vi "Parse CSV String.vi"(7 "delimiter (,)":string=",", 10 "error in":errorcluster, 11 "CSV string":string) -> (2 "error out":errorcluster, 3 "2-D array":string[][](array[string]))   [LabVIEW 2020, in "infolib.lvlib"]
doc: "<b>http://en.wikipedia.org/wiki/Comma-separated_values</b>\n\nConvert a CSV (Character Separated Values) spreadsheet string to a 2D array of strings.\nThe input CSV spreadsheet string is assumed to be ANSI encoded and formatted in accordance with RFC-4180 (see <b>http://tools.ietf.org/html/rfc4180</b>). \nAll escaped double quotes will be un-escaped in the output array.\n\nRev. 0.4.0 2017-03-01 updated for infostr - removed replacing of EOLS by LF and opening/closing quotes by straight quotes\n\nRev 0.3.0 02/20/2014 Ryan Porter\n- Added feature to replace all EOLs (0x0A, 0x0D) with LF (0x0A) so as to avoid adding a blank row when encountering CR+LF at the end of a line.\n- Added feature to allow any single character delimiter (not just the comma).\n- Removed the read text file and path terminals. \n- Changed Icon and connector pane layout.\n- Added error case structure around diagram.\n- Changed file name to Parse CSV String\n\nRev 0.2.0 06/08/2011 P. Brooks\n Added feature to replace opening and closing double quotes (0x93 & 0x94) with simple quote (0x22).\n\nRev 0.1.0 05/31/2011 P. Brooks\n Added option to handle strings. If CSV string is NULL (default) then the file in CSV File Path will be parsed instead of CSV string.\n\nRev 0.0.0 05/09/2011 P. Brooks\n Originated."
uses:
  infolib.lvlib
  <vilib>/Utility/error.llb/whitespace.ctl
panel:
  # "Parse CSV String.vi\n\nConvert a CSV (Character Separated Values) spreadsheet string to a 2D array of strings.\nThe input CSV spreadsheet string is assumed to be ANSI encoded and formatted in accordance with RFC-4180 (see http://tools.ietf.org/html/rfc4180). \nAll EOLs (CR, LF or CRLF) will be converted to LF and all escaped double quotes will be un-escaped in the output array."
  # "Wikipedia Example Text \n(using opening and closing quotes)"
  # "Year,Make,Model,Description,Price\n1997,Ford,E350, “ac, abs, moon”,3000.00\n1999,Chevy,“Venture ““Extended Edition”””,“”,4900.00\n1999,Chevy,“ Venture ““ Extended Edition, Very Large”””,“”,5000.00\n1996,Jeep,Grand Cherokee,“MUST SELL!\nair, moon roof, loaded”,4799.00"
  # "http://en.wikipedia.org/wiki/Comma-separated_values"
  # "Robust CSV v1.1.0\n\nCopyright © 2014, Ryan Porter\nAll rights reserved.\n\nAuthor:\t Ryan Porter\nLAVA Name: Porter\nContact Info:\tContact via PM on lavag.org\n\nLabVIEW Versions:\nLV 2013 (Windows)\nLV 2012 (Windows)\nLV 8.6 (Windows)\n\nDependencies:\nLAVA Palette\n\nDescription:\nThis package contains VIs for reading and writing to CSV files that follow the CSV format outlined in RFC-4180 (see http://tools.ietf.org/html/rfc4180). Using this package, you can properly import CSV files that were exported from spreadsheet programs such as Microsoft Excel, Open Office or LibreOffice Calc as well as export CSV files that will be compatible with any program capable of interpreting CSV files.\n \nThis implementation of the CSV format is capable of handling escaped fields such as those containing commas (or other field delimiters), multiple lines, and double quotes.\n\nInstallation and instructions:\nInstall VIP package using JKI VI Package Manager.\n\nExamples:\n\"<LabVIEW>\\examples\\LAVA\\Robust CSV\\Robust CSV Example Usage.vi\"\tDemonstrates usage of the Read CSV and Write CSV file.\n\nKnown Issues:\nnone\n\nAcknowledgements:\nPhillip Brooks: \"Parse CSV String.vi\" is a modified version of his \"CSV Data File Parser.vi\". His method of parsing the CSV string was much more efficient than my original implementation.\n\nVersion History:\nv1.0.0: Initial release of the code.\nv1.0.1: Modified \"Flatten to CSV Record.vi\" to play nice with Excel CSV import when multi-line cells are present.\nv1.1.0: Moved to LAVA palette & built to VI package file.\n\nLicense:\nDistributed under the BSD 2-Clause (http://opensource.org/licenses/BSD-2-Clause)\nSee link for a full description of the license.\n\nSupport:\nIf you have any problems with this code or want to suggest features go to lavag.org and Navigate to LAVA > Resources > Code Repository (Certified) and\nsearch for the \"Robust CSV\" support page. Or try this link: http://lavag.org/files/file/239-robust-csv/\n\nDistribution:\nThis code was downloaded from the LAVA Code Repository found at lavag.org"
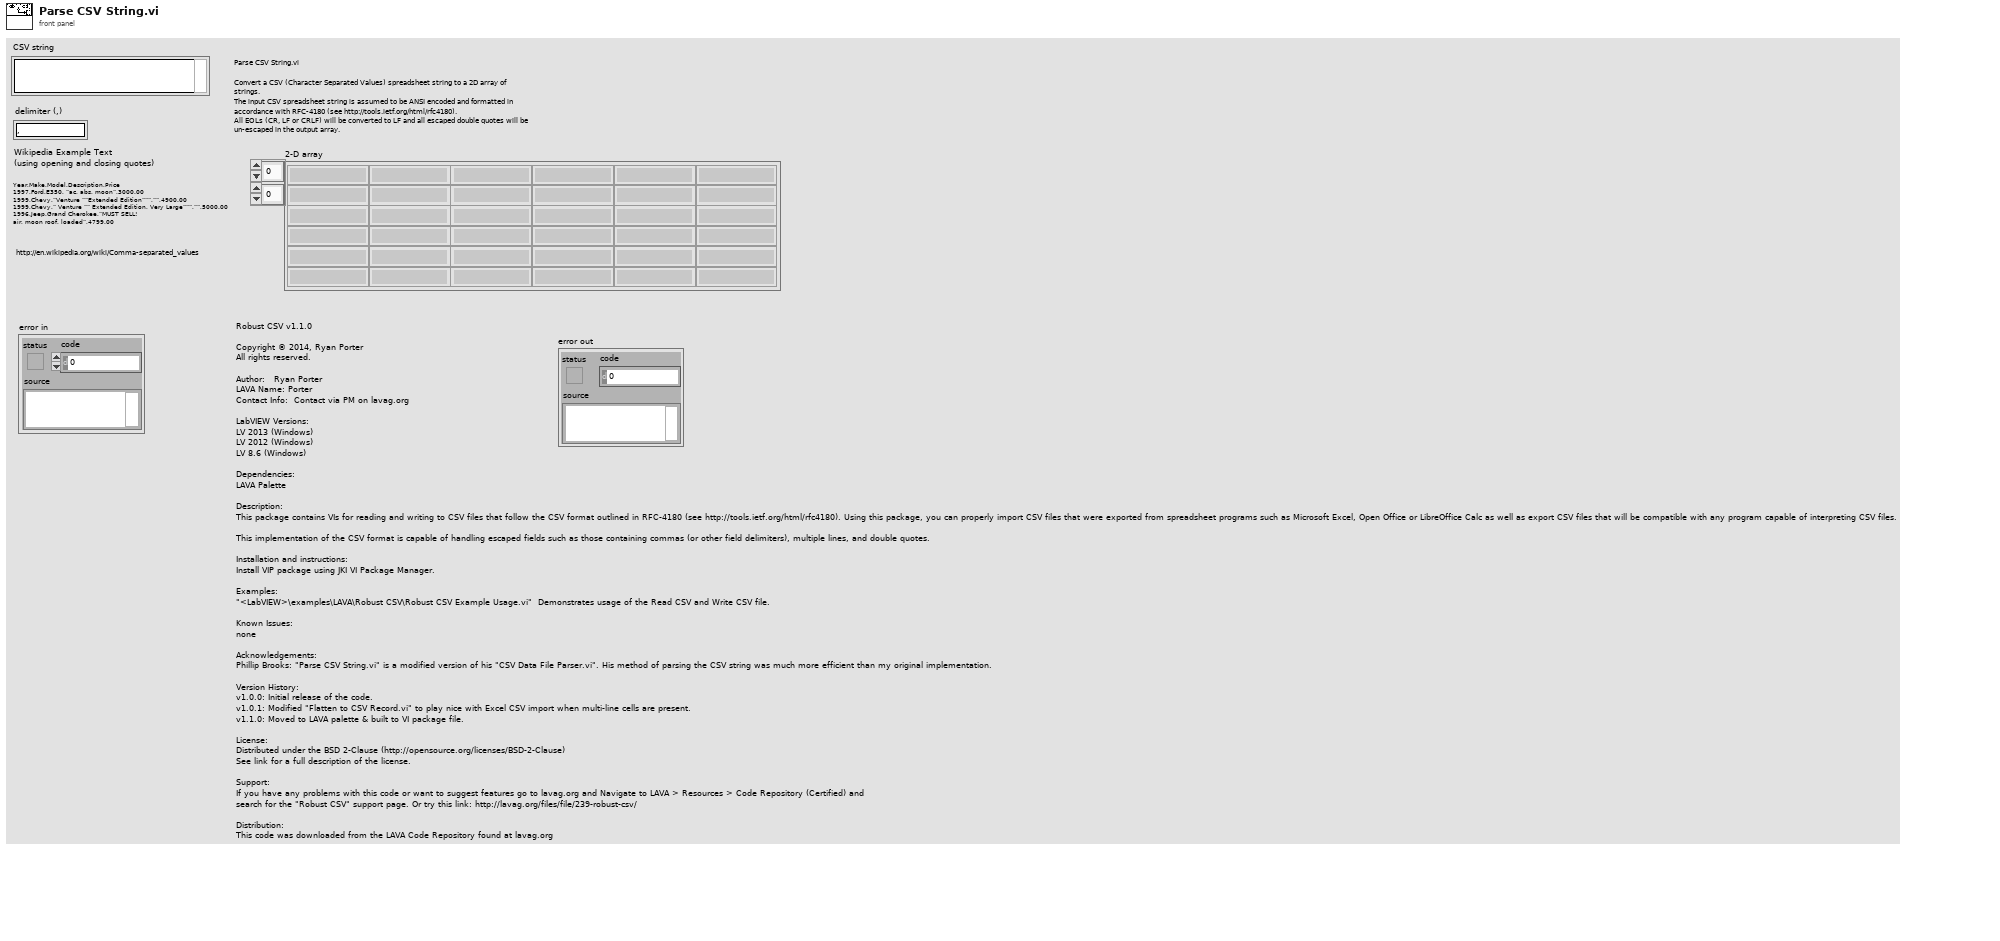
[diagram p1: front panel]
types:
  T1 = typedef "whitespace.ctl" = u16
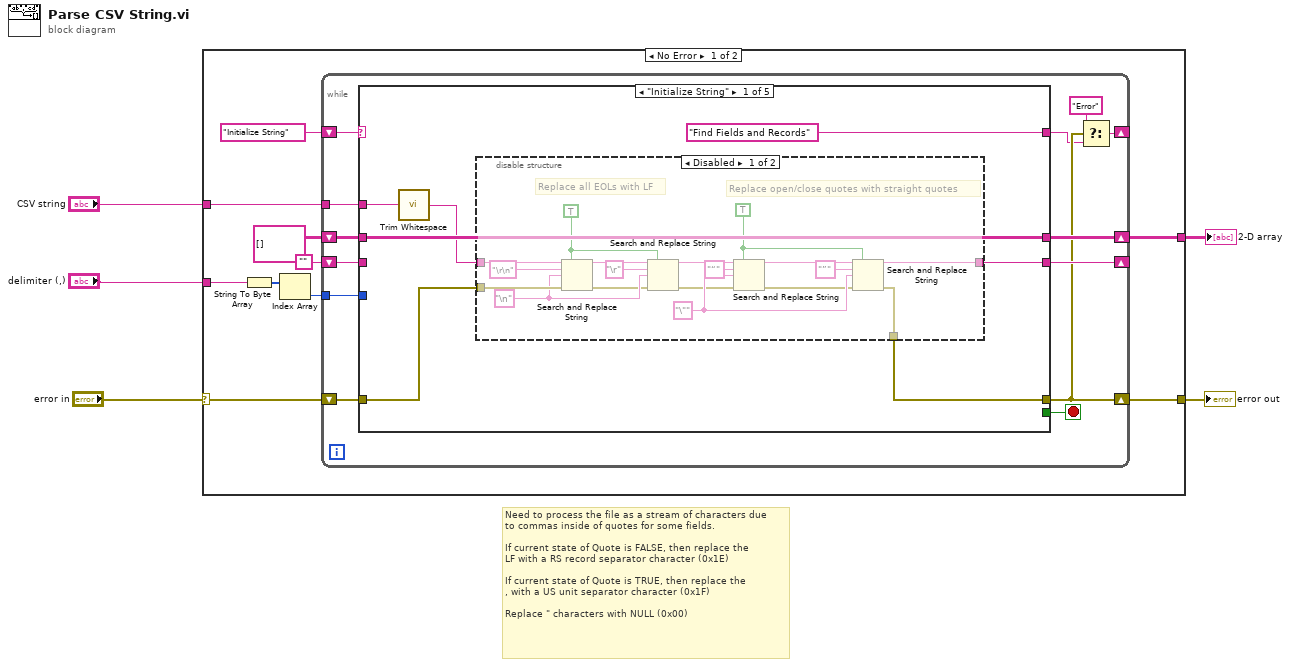
[diagram p0: block diagram]
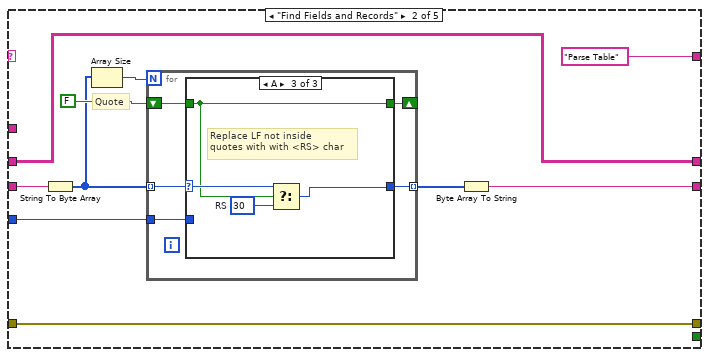
[diagram p3: hidden frame]
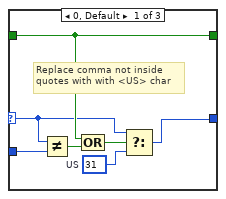
[diagram p4: hidden frame]
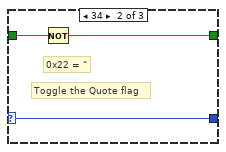
[diagram p5: hidden frame]
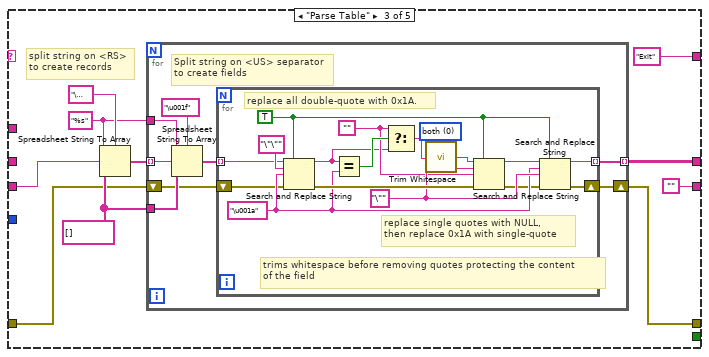
[diagram p6: hidden frame]
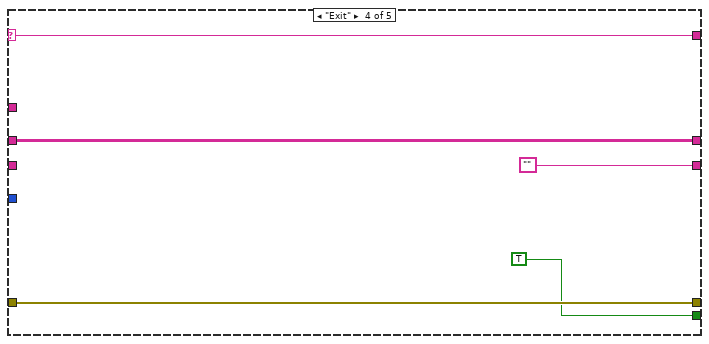
[diagram p7: hidden frame]
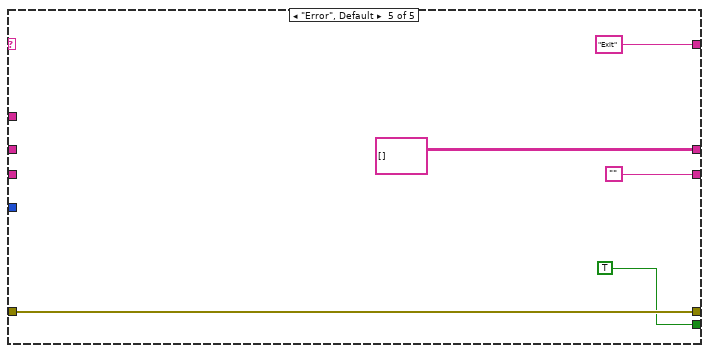
[diagram p8: hidden frame]
diagram:
  # "Need to process the file as a stream of characters due \nto commas inside of quotes for some fields.\n\nIf current state of Quote is FALSE, then replace the\nLF with a RS record separator character (0x1E)\n\nIf current state of Quote is TRUE, then replace the\n, with a US unit separator character (0x1F)\n\nReplace \" characters with NULL (0x00)"
  n1 = case shown="No Error" "error in" {
    selector: "error in" -> [w6 w130]
    tunnel: [w12 w130] -> w5
    tunnel: [w11 _] -> w4
    tunnel: "CSV string" -> [w10 _]
    tunnel: "delimiter (,)" -> [w9 _]
    frame No Error {
      n2 = String To Byte Array(string=w9) -> (unsigned byte array=w8:u8[])
      n3 = Index Array(array=w8) -> (element=w7:u8)  [unwired: 1 in]
      n4 = while {
        shift-right: [w28] -> _
        shift-left: "" -> [w27]
        shift-right: [w19] -> _
        shift-left: "Initialize String" -> [w24]
        shift-right: [w26] -> w11
        shift-left: string[][] [] -> [w25]
        shift-right: [w22] -> w12
        shift-left: w6 -> [w23]
        tunnel: w10 -> [w17]
        tunnel: w7 -> [w16]
        stop <- w18 stop-if-true
        n5 = case shown="\"Initialize String\"" w24 {
          selector: w24 -> [_ _ _ w123 _]
          tunnel: [w30 w60 "" "" ""] -> w28
          tunnel: ["Find Fields and Records" "Parse Table" "Exit" ("t") w123 "Exit" ("t")] -> w21
          tunnel: [_ _ _ TRUE TRUE] -> w18
          tunnel: w27 -> [_ w58 w86 _ _]
          tunnel: [w33 w59 w91 w120 string[][] []] -> w26
          tunnel: w25 -> [w33 w59 _ w120 _]
          tunnel: [w29 w56 w88 w124 w129] -> w22
          tunnel: w23 -> [w35 w56 w85 w124 w129]
          tunnel: w17 -> [w32 _ _ _ _]
          tunnel: w16 -> [_ w57 _ _ _]
          frame "Initialize String" {
            n6 = call <vilib>:"Trim Whitespace.vi"("string"=w32) -> ("trimmed string"=w31:string)  [unwired: 1 in]
            n7 = disable-structure shown="Disabled" {
              disable-tunnel: w35 -> [w53 w55]
              disable-tunnel: w31 -> [w52 w54]
              disable-tunnel: [w45 w54] -> w30
              disable-tunnel: [w43 w55] -> w29
              frame Disabled {
                w39 = TRUE ("replace all? (F)")
                w38 = "\n" ("search string")
                w46 = TRUE ("replace all? (F)")
                w48 = "\"" ("replace string (\"\")")
                # "Replace open/close quotes with straight quotes"
                # "Replace all EOLs with LF"
                n8 = Search and Replace String(replace all?=w39, input string=w52, search string="\r\n", replace string=w38, error in=w53) -> (result string=w41:string, error out=w36:errorcluster)  [unwired: 5 out]
                n9 = Search and Replace String(replace all?=w39, input string=w41, search string="\r", replace string=w38, error in=w36) -> (result string=w51:string, error out=w42:errorcluster)  [unwired: 5 out]
                n10 = Search and Replace String(replace all?=w46, input string=w51, search string="“", replace string=w48, error in=w42) -> (result string=w49:string, error out=w44:errorcluster)  [unwired: 5 out]
                n11 = Search and Replace String(replace all?=w46, input string=w49, search string="”", replace string=w48, error in=w44) -> (result string=w45:string, error out=w43:errorcluster)  [unwired: 5 out]
              }
              frame Enabled {
              }
            }
          }
          frame "Find Fields and Records" {
            # "Quote"
            n12 = String To Byte Array(string=w58) -> (unsigned byte array=w63:u8[])
            n13 = Array Size(array=w63) -> (size(s)=w64:i32)
            n14 = for {
              N: w64 -> [_]
              tunnel: w63 -> [w68] mode=indexing
              shift-right: [w69] -> _
              shift-left: FALSE -> [w70]
              tunnel: [w67] -> w61 mode=indexing
              tunnel: w57 -> [w66]
              n15 = case shown="A" w68 {
                selector: w68 -> [w71 w78 w82]
                tunnel: w70 -> [w74 w80 w81]
                tunnel: w66 -> [w76 _ _]
                tunnel: [w74 w79 w81] -> w69
                tunnel: [w77 w78 w83] -> w67
                frame 0, Default {
                  w72 = u8 31  # US
                  # "Replace comma not inside \nquotes with with <US> char"
                  n16 = Not Equal?(x=w71, y=w76) -> (x != y?=w75:bool)
                  n17 = Compound Arithmetic op=OR(w74, w75) -> (w73:bool)
                  n18 = Select(t=w71, s=w73, f=w72) -> (s? t:f=w77:u8)
                }
                frame 34 {
                  # "0x22 = \""
                  # "Toggle the Quote flag"
                  n19 = Not(x=w80) -> (.not. x?=w79:bool)
                }
                frame 10 {
                  w84 = u8 30  # RS
                  # "Replace LF not inside \nquotes with with <RS> char"
                  n20 = Select(t=w82, s=w81, f=w84) -> (s? t:f=w83:u8)
                }
              }
            }
            n21 = Byte Array To String(unsigned byte array=w61) -> (string=w60:string)
          }
          frame "Parse Table" {
            w94 = string[] []
            w89 = "%s" ("format string")
            # "split string on <RS>\nto create records"
            n22 = Spreadsheet String To Array(delimiter (Tab)="\u001e", format string=w89, spreadsheet string=w86, array type (2D Dbl)=w94) -> (array=w93:string[])
            n23 = for {
              tunnel: w93 -> [w102] mode=indexing
              tunnel: w94 -> [w99]
              tunnel: [w98] -> w91 mode=indexing
              tunnel: w89 -> [w97]
              shift-right: [w95] -> w88
              shift-left: w85 -> [w96]
              # "Split string on <US> separator\nto create fields"
              n24 = Spreadsheet String To Array(delimiter (Tab)="\u001f", format string=w97, spreadsheet string=w102, array type (2D Dbl)=w99) -> (array=w100:string[])
              n25 = for {
                tunnel: w100 -> [w106] mode=indexing
                tunnel: [w107] -> w98 mode=indexing
                shift-right: [w108] -> w95
                shift-left: w96 -> [w110]
                w103 = T1 0 items=["both", "start of string", "end of string"] ("location (both)")
                w112 = ""
                w115 = "\"" ("input string")
                w116 = TRUE ("replace all? (F)")
                w114 = "\u001a" ("replace string (\"\")")
                # "trims whitespace before removing quotes protecting the content\nof the field"
                # "replace single quotes with NULL,\nthen replace 0x1A with single-quote"
                # "replace all double-quote with 0x1A."
                n26 = Search and Replace String(replace all?=w116, input string=w106, search string="\"\"", replace string=w114, error in=w110) -> (result string=w111:string, error out=w118:errorcluster)  [unwired: 5 out]
                n27 = Equal?(x=w111, y=w114) -> (x = y?=w113:bool)
                n28 = Select(t=w112, s=w113, f=w111) -> (s? t:f=w105:string)
                n29 = call <vilib>:"Trim Whitespace.vi"("string"=w105, "location (both)"=w103) -> ("trimmed string"=w104:string)
                n30 = Search and Replace String(replace all?=w116, input string=w104, search string=w115, replace string=w112, error in=w118) -> (result string=w117:string, error out=w109:errorcluster)  [unwired: 5 out]
                n31 = Search and Replace String(replace all?=w116, input string=w117, search string=w114, replace string=w115, error in=w109) -> (result string=w107:string, error out=w108:errorcluster)  [unwired: 1 in, 4 out]
              }
            }
          }
          frame "Exit" {
          }
          frame "Error", Default {
          }
        }
        n32 = Select(t="Error", s=w22, f=w21) -> (s? t:f=w19:string)
      }
    }
    frame Error {
    }
  }
  "error out" <- w5
  "2-D array" <- w4
